vi "Eurotherm_New_Module.vi"(4 "Decimales":u16(ring)=1 items=["0"=1, "1"=10, "2"=100], 5 "Eurotherm (T:Enable)":bool=TRUE, 7 "Command":T3, 8 "error in (no error)":errorcluster, 9 "Value":dbl format="%04.1g", 10 "Address":T2(ring), 11 "VISA resource name":refnum<visa-resource-name>) -> (0 "error out":errorcluster, 2 "Eurotherm":T1)   [LabVIEW 2017]
uses:
  Eurotherm_New_Module.ctl
  <vilib>/Instr/_visa.llb/VISA Configure Serial Port (Instr).vi
panel:
  out "String Read":string
  out "String Write":string
  # "Eurotherm New Module"
  # "Input Data"
  # "Local Data"
  # "Output Data"
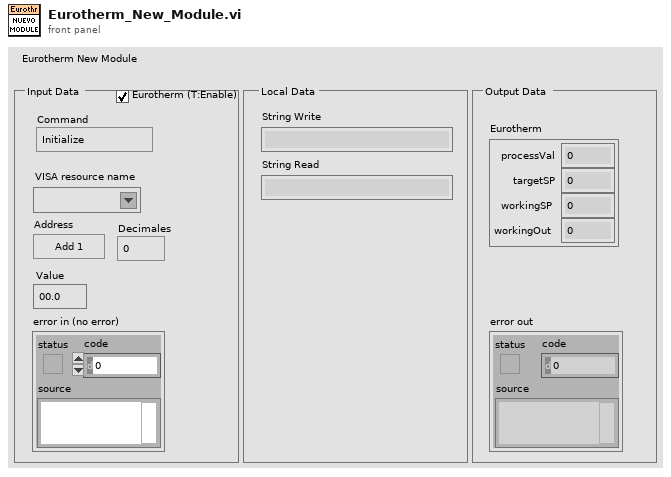
[diagram p1: front panel]
types:
  T1 = cluster{"processVal":dbl, "targetSP":dbl, "workingSP":dbl, "workingOut":dbl}
  T2 = enum16{"Add 1", "Add 2", "Add 10", "Add 11", "Add 12", "Add 13"}
  T3 = typedef "Eurotherm_New_Module.ctl" = enum16{"Initialize", "Write SP", "Read SP+PV", "Write Rate", "Set P", "Set I", "Set D", "Shutdown"}
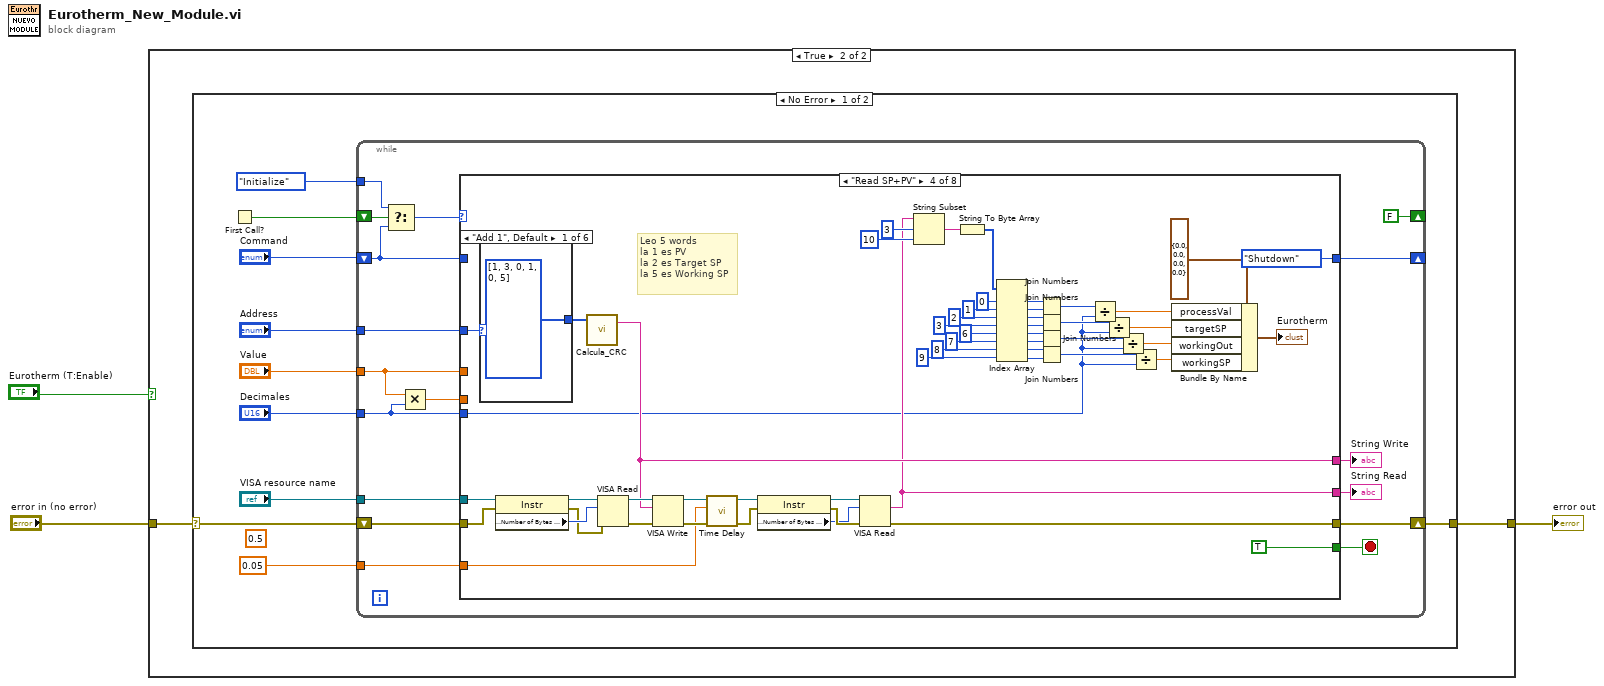
[diagram p0: block diagram]
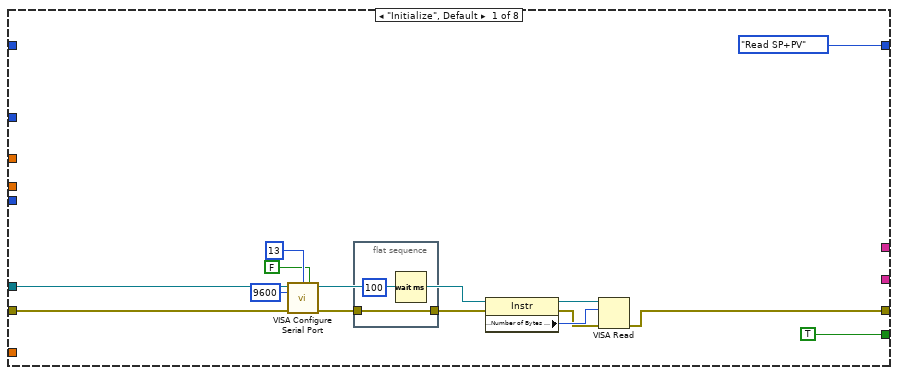
[diagram p3: hidden frame]
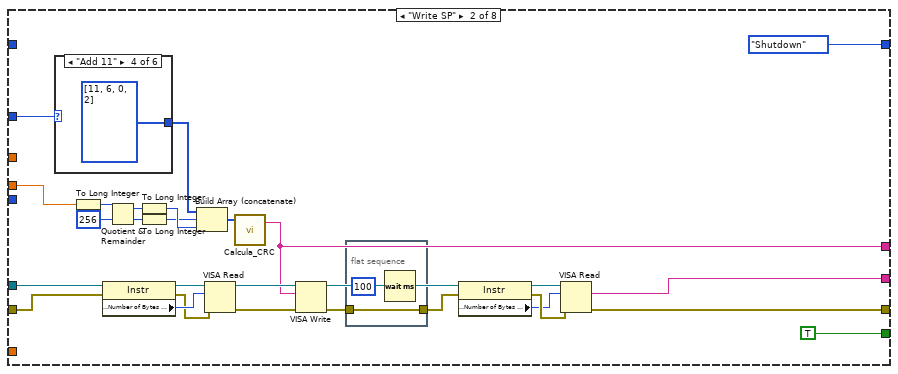
[diagram p4: hidden frame]
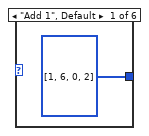
[diagram p5: hidden frame]
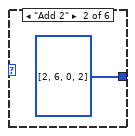
[diagram p6: hidden frame]
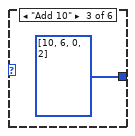
[diagram p7: hidden frame]
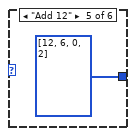
[diagram p8: hidden frame]
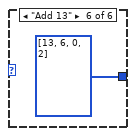
[diagram p9: hidden frame]
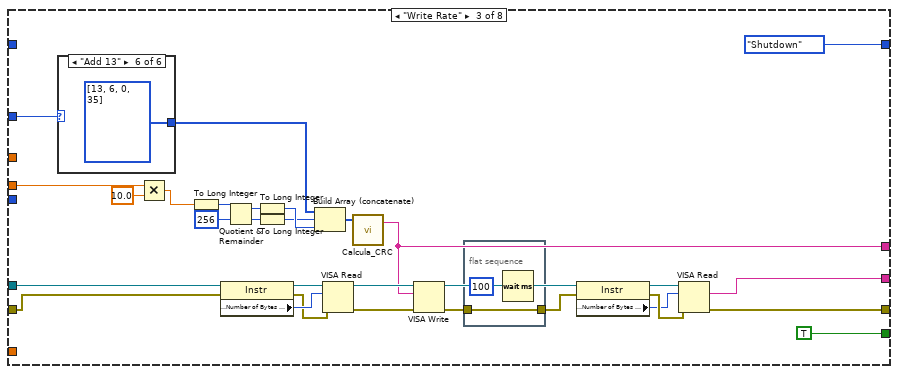
[diagram p10: hidden frame]
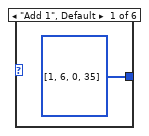
[diagram p11: hidden frame]
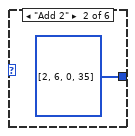
[diagram p12: hidden frame]
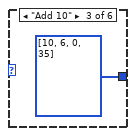
[diagram p13: hidden frame]
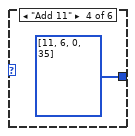
[diagram p14: hidden frame]
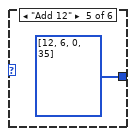
[diagram p15: hidden frame]
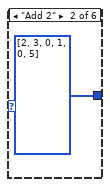
[diagram p16: hidden frame]
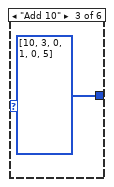
[diagram p17: hidden frame]
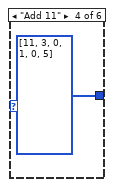
[diagram p18: hidden frame]
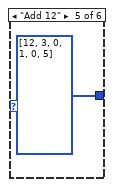
[diagram p19: hidden frame]
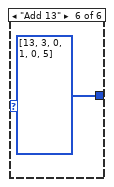
[diagram p20: hidden frame]
diagram:
  n1 = case shown="True" "Eurotherm (T:Enable)" {
    tunnel: "error in (no error)" -> [w4 w6]
    tunnel: [w4 w5] -> w2
    frame False {
    }
    frame True {
      n2 = case shown="No Error" w6 {
        selector: w6 -> [w14 w295]
        tunnel: [w13 w295] -> w5
        frame No Error {
          (unwired) 0.5 ("milliseconds to wait")
          n3 = First Call?() -> (First Call?: T/F=w16:bool)
          n4 = while {
            shift-right: [w28] -> _
            shift-left: "Command" -> [w29]
            shift-right: [w26] -> w13
            shift-left: w14 -> [w25]
            shift-right: [FALSE ("First Call?: T/F")] -> _
            shift-left: w16 -> [w33]
            tunnel: Eurotherm_New_Module."Initialize" ("t") -> [w32]
            tunnel: "Address" -> [w22]
            tunnel: "Value" -> [w19]
            tunnel: "Decimales" -> [w21]
            tunnel: "VISA resource name" -> [w18]
            tunnel: 0.05 ("milliseconds to wait") -> [w17]
            stop <- w27 stop-if-true
            n5 = Select(t=w32, s=w33, f=w29) -> (s? t:f=w30:T3)
            n6 = Multiply(x=w19, y=w21) -> (x*y=w20:dbl)
            n7 = case shown="\"Read SP+PV\"" w30 {
              tunnel: w29 -> [_ _ _ _ _ _ _ _]
              tunnel: [Eurotherm_New_Module."Read SP+PV" ("s? t:f") Eurotherm_New_Module."Shutdown" ("s? t:f") Eurotherm_New_Module."Shutdown" ("s? t:f") Eurotherm_New_Module."Shutdown" ("s? t:f") Eurotherm_New_Module."Shutdown" ("s? t:f") Eurotherm_New_Module."Shutdown" ("s? t:f") Eurotherm_New_Module."Shutdown" ("s? t:f") Eurotherm_New_Module."Shutdown" ("s? t:f")] -> w28
              tunnel: [TRUE ("First Call?: T/F") TRUE ("First Call?: T/F") TRUE ("First Call?: T/F") TRUE ("First Call?: T/F") TRUE ("First Call?: T/F") TRUE ("First Call?: T/F") TRUE ("First Call?: T/F") TRUE ("First Call?: T/F")] -> w27
              tunnel: [w37 w57 w91 w152 w189 w225 w261 w290] -> w26
              tunnel: w25 -> [w38 w58 w95 w164 w190 w226 w262 w291]
              tunnel: w18 -> [w34 w56 w96 w163 w188 w224 w260 w292]
              tunnel: [_ w55 w90 w153 w187 w223 w259 _] -> w24
              tunnel: [_ w54 w89 w162 w186 w222 w258 _] -> w23
              tunnel: w22 -> [_ w51 w94 w175 w183 w219 w255 _]
              tunnel: w20 -> [_ w50 w88 _ _ _ _ _]
              tunnel: w21 -> [_ _ _ w130 _ _ _ _]
              tunnel: w19 -> [_ _ _ _ w182 w218 w254 _]
              tunnel: w17 -> [_ _ _ w139 _ _ _ _]
              frame "Initialize", Default {
                n8 = call-poly "VISA Configure Serial Port"("VISA resource name"=w34, "termination char\n(0xA = '\\n' = LF)"=u8 13 ("termination char\n(0xA = '\\n' = LF)"), "Enable Termination\nChar (T)"=FALSE ("Enable Termination\nChar (T)"), "baud rate (9600)"=u32 9600, "error in (no error)"=w38) -> ("VISA resource name out"=w39:refnum<visa-resource-name>, "error out"=w40:errorcluster)  [unwired: 9 in]
                n9 = flat-sequence {
                  tunnel: w40 -> [w48]
                  tunnel: [w48] -> w47
                  frame #0 {
                    n10 = Wait (ms)(milliseconds to wait=u32 100) -> ()  [unwired: 1 out]
                  }
                }
                n11 = property class="Instr"(reference=w39, error in=w47) -> (reference out=w44:refnum<visa-resource-name>, error out=w45:errorcluster, "Serial Settings:Number of Bytes at Serial Port"=w46:u32)
                n12 = VISA Read(VISA resource name=w44, byte count=w46, error in (no error)=w45) -> (error out=w37:errorcluster)  [unwired: 3 out]
              }
              frame "Write SP" {
                n13 = case shown="\"Add 11\"" w51 {
                  tunnel: [u8[] [1, 6, 0, 2] ("Message Data") u8[] [2, 6, 0, 2] ("Message Data") u8[] [10, 6, 0, 2] ("Message Data") u8[] [11, 6, 0, 2] ("Message Data") u8[] [12, 6, 0, 2] ("Message Data") u8[] [13, 6, 0, 2] ("Message Data")] -> w77
                  frame "Add 1", Default {
                  }
                  frame "Add 2" {
                  }
                  frame "Add 10" {
                  }
                  frame "Add 11" {
                  }
                  frame "Add 12" {
                  }
                  frame "Add 13" {
                  }
                }
                n14 = To Long Integer(number=w50) -> (32bit integer=w76:i32)
                n15 = property class="Instr"(reference=w56, error in=w58) -> (reference out=w59:refnum<visa-resource-name>, error out=w60:errorcluster, "Serial Settings:Number of Bytes at Serial Port"=w61:u32)
                n16 = Quotient & Remainder(x=w76, y=256) -> (x-y*floor(x/y)=w71:i32, floor(x/y)=w72:i32)
                n17 = To Long Integer(number=w71) -> (32bit integer=w74:i32)
                n18 = To Long Integer(number=w72) -> (32bit integer=w73:i32)
                n19 = Build Array (concatenate)(w77, w73, w74) -> (w75:i32[])
                n20 = VISA Read(VISA resource name=w59, byte count=w61, error in (no error)=w60) -> (VISA resource name out=w68:refnum<visa-resource-name>, error out=w67:errorcluster)  [unwired: 2 out]
                n21 = call "Calcula_CRC.vi"("Message Data"=w75) -> ("String"=w54:string)  [unwired: 2 in, 1 out]
                n22 = VISA Write(VISA resource name=w68, write buffer=w54, error in (no error)=w67) -> (VISA resource name out=w69:refnum<visa-resource-name>, error out=w66:errorcluster)  [unwired: 1 out]
                n23 = flat-sequence {
                  tunnel: w66 -> [w78]
                  tunnel: [w78] -> w65
                  frame #0 {
                    n24 = Wait (ms)(milliseconds to wait=u32 100) -> ()  [unwired: 1 out]
                  }
                }
                n25 = property class="Instr"(reference=w69, error in=w65) -> (reference out=w64:refnum<visa-resource-name>, error out=w63:errorcluster, "Serial Settings:Number of Bytes at Serial Port"=w62:u32)
                n26 = VISA Read(VISA resource name=w64, byte count=w62, error in (no error)=w63) -> (read buffer=w55:string, error out=w57:errorcluster)  [unwired: 2 out]
              }
              frame "Write Rate" {
                n27 = case shown="\"Add 13\"" w94 {
                  tunnel: [u8[] [1, 6, 0, 35] ("Message Data") u8[] [2, 6, 0, 35] ("Message Data") u8[] [10, 6, 0, 35] ("Message Data") u8[] [11, 6, 0, 35] ("Message Data") u8[] [12, 6, 0, 35] ("Message Data") u8[] [13, 6, 0, 35] ("Message Data")] -> w115
                  frame "Add 1", Default {
                  }
                  frame "Add 2" {
                  }
                  frame "Add 10" {
                  }
                  frame "Add 11" {
                  }
                  frame "Add 12" {
                  }
                  frame "Add 13" {
                  }
                }
                n28 = Multiply(x=w88, y=10.0) -> (x*y=w87:dbl)
                n29 = To Long Integer(number=w87) -> (32bit integer=w114:i32)
                n30 = property class="Instr"(reference=w96, error in=w95) -> (reference out=w97:refnum<visa-resource-name>, error out=w98:errorcluster, "Serial Settings:Number of Bytes at Serial Port"=w99:u32)
                n31 = Quotient & Remainder(x=w114, y=256) -> (x-y*floor(x/y)=w109:i32, floor(x/y)=w110:i32)
                n32 = To Long Integer(number=w109) -> (32bit integer=w112:i32)
                n33 = To Long Integer(number=w110) -> (32bit integer=w111:i32)
                n34 = Build Array (concatenate)(w115, w111, w112) -> (w113:i32[])
                n35 = VISA Read(VISA resource name=w97, byte count=w99, error in (no error)=w98) -> (VISA resource name out=w106:refnum<visa-resource-name>, error out=w105:errorcluster)  [unwired: 2 out]
                n36 = call "Calcula_CRC.vi"("Message Data"=w113) -> ("String"=w89:string)  [unwired: 2 in, 1 out]
                n37 = VISA Write(VISA resource name=w106, write buffer=w89, error in (no error)=w105) -> (VISA resource name out=w107:refnum<visa-resource-name>, error out=w104:errorcluster)  [unwired: 1 out]
                n38 = flat-sequence {
                  tunnel: w104 -> [w116]
                  tunnel: [w116] -> w103
                  frame #0 {
                    n39 = Wait (ms)(milliseconds to wait=u32 100) -> ()  [unwired: 1 out]
                  }
                }
                n40 = property class="Instr"(reference=w107, error in=w103) -> (reference out=w102:refnum<visa-resource-name>, error out=w101:errorcluster, "Serial Settings:Number of Bytes at Serial Port"=w100:u32)
                n41 = VISA Read(VISA resource name=w102, byte count=w100, error in (no error)=w101) -> (read buffer=w90:string, error out=w91:errorcluster)  [unwired: 2 out]
              }
              frame "Read SP+PV" {
                # "Leo 5 words\nla 1 es PV\nla 2 es Target SP\nla 5 es Working SP"
                n42 = case shown="\"Add 1\", Default" w175 {
                  tunnel: [u8[] [1, 3, 0, 1, 0, 5] ("Message Data") u8[] [2, 3, 0, 1, 0, 5] ("Message Data") u8[] [10, 3, 0, 1, 0, 5] ("Message Data") u8[] [11, 3, 0, 1, 0, 5] ("Message Data") u8[] [12, 3, 0, 1, 0, 5] ("Message Data") u8[] [13, 3, 0, 1, 0, 5] ("Message Data")] -> w174
                  frame "Add 1", Default {
                  }
                  frame "Add 2" {
                  }
                  frame "Add 10" {
                  }
                  frame "Add 11" {
                  }
                  frame "Add 12" {
                  }
                  frame "Add 13" {
                  }
                }
                n43 = property class="Instr"(reference=w163, error in=w164) -> (reference out=w165:refnum<visa-resource-name>, error out=w166:errorcluster, "Serial Settings:Number of Bytes at Serial Port"=w167:u32)
                n44 = call "Calcula_CRC.vi"("Message Data"=w174) -> ("String"=w162:string)  [unwired: 2 in, 1 out]
                n45 = VISA Read(VISA resource name=w165, byte count=w167, error in (no error)=w166) -> (VISA resource name out=w172:refnum<visa-resource-name>, error out=w171:errorcluster)  [unwired: 2 out]
                n46 = VISA Write(VISA resource name=w172, write buffer=w162, error in (no error)=w171) -> (VISA resource name out=w173:refnum<visa-resource-name>, error out=w141:errorcluster)  [unwired: 1 out]
                n47 = call "Time Delay"("error in (no error)"=w141, "Delay Time (s)"=w139) -> ("error out"=w140:errorcluster)  [unwired: 9 in]
                n48 = property class="Instr"(reference=w173, error in=w140) -> (reference out=w170:refnum<visa-resource-name>, error out=w169:errorcluster, "Serial Settings:Number of Bytes at Serial Port"=w168:u32)
                n49 = VISA Read(VISA resource name=w170, byte count=w168, error in (no error)=w169) -> (read buffer=w153:string, error out=w152:errorcluster)  [unwired: 2 out]
                n50 = String Subset(string=w153, offset (0)=3, length (rest)=10 ("length (rest)")) -> (substring=w154:string)
                n51 = String To Byte Array(string=w154) -> (unsigned byte array=w157:u8[])
                n52 = Index Array(array=w157, index #1=0 ("index"), index #2=1 ("index"), index #3=2 ("index"), index #4=3 ("index"), index #5=6 ("index"), index #6=7 ("index"), index #7=8 ("index"), index #8=9 ("index")) -> (element #1=w145:u8, element #2=w144:u8, element #3=w143:u8, element #4=w142:u8, element #5=w138:u8, element #6=w137:u8, element #7=w136:u8, element #8=w135:u8)
                n53 = Join Numbers(hi=w145, lo=w144) -> ((hi.lo)=w134:u16)
                n54 = Join Numbers(hi=w143, lo=w142) -> ((hi.lo)=w133:u16)
                n55 = Join Numbers(hi=w138, lo=w137) -> ((hi.lo)=w132:u16)
                n56 = Join Numbers(hi=w136, lo=w135) -> ((hi.lo)=w131:u16)
                n57 = Divide(x=w134, y=w130) -> (x/y=w125:dbl)
                n58 = Divide(x=w133, y=w130) -> (x/y=w126:dbl)
                n59 = Divide(x=w132, y=w130) -> (x/y=w127:dbl)
                n60 = Divide(x=w131, y=w130) -> (x/y=w128:dbl)
                n61 = Bundle By Name(cluster=T1 {"processVal"=0.0, "targetSP"=0.0, "workingSP"=0.0, "workingOut"=0.0} ("Eurotherm"), "processVal"=w125, "targetSP"=w126, "workingOut"=w127, "workingSP"=w128) -> (→"Eurotherm":T1)
              }
              frame "Set P" {
                n62 = case shown="\"Add 1\", Default" w183 {
                  tunnel: [u8[] [1, 6, 0, 6] ("Message Data") u8[] [2, 6, 0, 6] ("Message Data") u8[] [10, 6, 0, 6] ("Message Data") u8[] [11, 6, 0, 6] ("Message Data") u8[] [12, 6, 0, 6] ("Message Data") u8[] [13, 6, 0, 6] ("Message Data")] -> w209
                  frame "Add 1", Default {
                  }
                  frame "Add 2" {
                  }
                  frame "Add 10" {
                  }
                  frame "Add 11" {
                  }
                  frame "Add 12" {
                  }
                  frame "Add 13" {
                  }
                }
                n63 = To Long Integer(number=w182) -> (32bit integer=w208:i32)
                n64 = property class="Instr"(reference=w188, error in=w190) -> (reference out=w191:refnum<visa-resource-name>, error out=w192:errorcluster, "Serial Settings:Number of Bytes at Serial Port"=w193:u32)
                n65 = Quotient & Remainder(x=w208, y=256) -> (x-y*floor(x/y)=w203:i32, floor(x/y)=w204:i32)
                n66 = To Long Integer(number=w203) -> (32bit integer=w206:i32)
                n67 = To Long Integer(number=w204) -> (32bit integer=w205:i32)
                n68 = Build Array (concatenate)(w209, w205, w206) -> (w207:i32[])
                n69 = VISA Read(VISA resource name=w191, byte count=w193, error in (no error)=w192) -> (VISA resource name out=w200:refnum<visa-resource-name>, error out=w199:errorcluster)  [unwired: 2 out]
                n70 = call "Calcula_CRC.vi"("Message Data"=w207) -> ("String"=w186:string)  [unwired: 2 in, 1 out]
                n71 = VISA Write(VISA resource name=w200, write buffer=w186, error in (no error)=w199) -> (VISA resource name out=w201:refnum<visa-resource-name>, error out=w198:errorcluster)  [unwired: 1 out]
                n72 = flat-sequence {
                  tunnel: w198 -> [w210]
                  tunnel: [w210] -> w197
                  frame #0 {
                    n73 = Wait (ms)(milliseconds to wait=u32 100) -> ()  [unwired: 1 out]
                  }
                }
                n74 = property class="Instr"(reference=w201, error in=w197) -> (reference out=w196:refnum<visa-resource-name>, error out=w195:errorcluster, "Serial Settings:Number of Bytes at Serial Port"=w194:u32)
                n75 = VISA Read(VISA resource name=w196, byte count=w194, error in (no error)=w195) -> (read buffer=w187:string, error out=w189:errorcluster)  [unwired: 2 out]
              }
              frame "Set I" {
                n76 = case shown="\"Add 13\"" w219 {
                  tunnel: [u8[] [1, 6, 0, 8] ("Message Data") u8[] [2, 6, 0, 8] ("Message Data") u8[] [10, 6, 0, 8] ("Message Data") u8[] [11, 6, 0, 8] ("Message Data") u8[] [12, 6, 0, 8] ("Message Data") u8[] [13, 6, 0, 8] ("Message Data")] -> w245
                  frame "Add 1", Default {
                  }
                  frame "Add 2" {
                  }
                  frame "Add 10" {
                  }
                  frame "Add 11" {
                  }
                  frame "Add 12" {
                  }
                  frame "Add 13" {
                  }
                }
                n77 = To Long Integer(number=w218) -> (32bit integer=w244:i32)
                n78 = property class="Instr"(reference=w224, error in=w226) -> (reference out=w227:refnum<visa-resource-name>, error out=w228:errorcluster, "Serial Settings:Number of Bytes at Serial Port"=w229:u32)
                n79 = Quotient & Remainder(x=w244, y=256) -> (x-y*floor(x/y)=w239:i32, floor(x/y)=w240:i32)
                n80 = To Long Integer(number=w239) -> (32bit integer=w242:i32)
                n81 = To Long Integer(number=w240) -> (32bit integer=w241:i32)
                n82 = Build Array (concatenate)(w245, w241, w242) -> (w243:i32[])
                n83 = VISA Read(VISA resource name=w227, byte count=w229, error in (no error)=w228) -> (VISA resource name out=w236:refnum<visa-resource-name>, error out=w235:errorcluster)  [unwired: 2 out]
                n84 = call "Calcula_CRC.vi"("Message Data"=w243) -> ("String"=w222:string)  [unwired: 2 in, 1 out]
                n85 = VISA Write(VISA resource name=w236, write buffer=w222, error in (no error)=w235) -> (VISA resource name out=w237:refnum<visa-resource-name>, error out=w234:errorcluster)  [unwired: 1 out]
                n86 = flat-sequence {
                  tunnel: w234 -> [w246]
                  tunnel: [w246] -> w233
                  frame #0 {
                    n87 = Wait (ms)(milliseconds to wait=u32 100) -> ()  [unwired: 1 out]
                  }
                }
                n88 = property class="Instr"(reference=w237, error in=w233) -> (reference out=w232:refnum<visa-resource-name>, error out=w231:errorcluster, "Serial Settings:Number of Bytes at Serial Port"=w230:u32)
                n89 = VISA Read(VISA resource name=w232, byte count=w230, error in (no error)=w231) -> (read buffer=w223:string, error out=w225:errorcluster)  [unwired: 2 out]
              }
              frame "Set D" {
                n90 = case shown="\"Add 13\"" w255 {
                  tunnel: [u8[] [1, 6, 0, 9] ("Message Data") u8[] [2, 6, 0, 9] ("Message Data") u8[] [10, 6, 0, 9] ("Message Data") u8[] [11, 6, 0, 9] ("Message Data") u8[] [12, 6, 0, 9] ("Message Data") u8[] [13, 6, 0, 9] ("Message Data")] -> w281
                  frame "Add 1", Default {
                  }
                  frame "Add 2" {
                  }
                  frame "Add 10" {
                  }
                  frame "Add 11" {
                  }
                  frame "Add 12" {
                  }
                  frame "Add 13" {
                  }
                }
                n91 = To Long Integer(number=w254) -> (32bit integer=w280:i32)
                n92 = property class="Instr"(reference=w260, error in=w262) -> (reference out=w263:refnum<visa-resource-name>, error out=w264:errorcluster, "Serial Settings:Number of Bytes at Serial Port"=w265:u32)
                n93 = Quotient & Remainder(x=w280, y=256) -> (x-y*floor(x/y)=w275:i32, floor(x/y)=w276:i32)
                n94 = To Long Integer(number=w275) -> (32bit integer=w278:i32)
                n95 = To Long Integer(number=w276) -> (32bit integer=w277:i32)
                n96 = Build Array (concatenate)(w281, w277, w278) -> (w279:i32[])
                n97 = VISA Read(VISA resource name=w263, byte count=w265, error in (no error)=w264) -> (VISA resource name out=w272:refnum<visa-resource-name>, error out=w271:errorcluster)  [unwired: 2 out]
                n98 = call "Calcula_CRC.vi"("Message Data"=w279) -> ("String"=w258:string)  [unwired: 2 in, 1 out]
                n99 = VISA Write(VISA resource name=w272, write buffer=w258, error in (no error)=w271) -> (VISA resource name out=w273:refnum<visa-resource-name>, error out=w270:errorcluster)  [unwired: 1 out]
                n100 = flat-sequence {
                  tunnel: w270 -> [w282]
                  tunnel: [w282] -> w269
                  frame #0 {
                    n101 = Wait (ms)(milliseconds to wait=u32 100) -> ()  [unwired: 1 out]
                  }
                }
                n102 = property class="Instr"(reference=w273, error in=w269) -> (reference out=w268:refnum<visa-resource-name>, error out=w267:errorcluster, "Serial Settings:Number of Bytes at Serial Port"=w266:u32)
                n103 = VISA Read(VISA resource name=w268, byte count=w266, error in (no error)=w267) -> (read buffer=w259:string, error out=w261:errorcluster)  [unwired: 2 out]
              }
              frame "Shutdown" {
                n104 = VISA Close(VISA resource name=w292, error in (no error)=w291) -> (error out=w290:errorcluster)
              }
            }
            "String Read" <- w24
            "String Write" <- w23
          }
        }
        frame Error {
        }
      }
    }
  }
  "error out" <- w2
